vi "Error Handler.vi"(8 "error in (no error)":errorcluster, 9 "Motor Error Status (none)":T1, 10 "Error? (no error)":bool, 11 "Error type":u16(ring) items=["Default (no error)", "Scan timeout", "Invalid motor checksum", "Unexpected return string", "Invalid address range"]) -> (0 "error out":errorcluster)   [LabVIEW 2012, in "Roboteq.lvlib"]
doc: "This VI defines the error codes used for the Dynamixel motor driver."
uses:
  Roboteq.lvlib
  <instrlib>/Dynamixel Motor/Public/Motor Operation/Low Level/Alarm Setting.ctl
  <instrlib>/Dynamixel Motor/Dynamixel Motor.lvlib
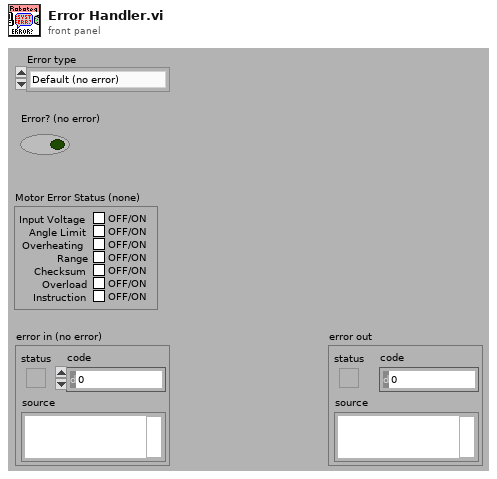
[diagram p1: front panel]
types:
  T1 = typedef "Dynamixel Motor.lvlib/Alarm Setting.ctl" = cluster{"Input Voltage":bool, "Angle Limit":bool, "Overheating ":bool, "Range":bool, "Checksum":bool, "Overload":bool, "Instruction":bool}
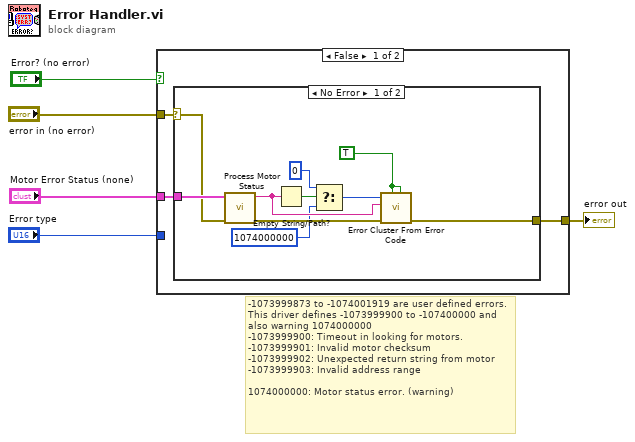
[diagram p0: block diagram]
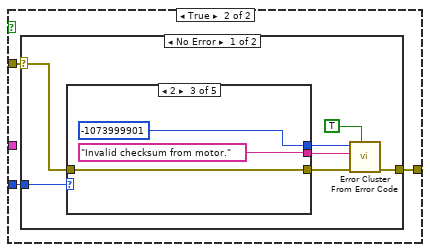
[diagram p3: hidden frame]
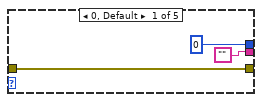
[diagram p4: hidden frame]
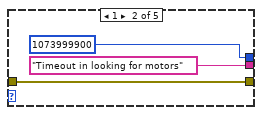
[diagram p5: hidden frame]
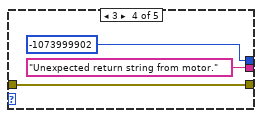
[diagram p6: hidden frame]
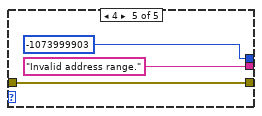
[diagram p7: hidden frame]
diagram:
  # "-1073999873 to -1074001919 are user defined errors.  This driver defines -1073999900 to -107400000 and also warning 1074000000\n-1073999900: Timeout in looking for motors.\n-1073999901: Invalid motor checksum\n-1073999902: Unexpected return string from motor\n-1073999903: Invalid address range\n\n1074000000: Motor status error. (warning)"
  n1 = case shown="False" "Error? (no error)" {
    tunnel: "error in (no error)" -> [w8 w22]
    tunnel: [w7 w21] -> w4
    tunnel: "Error type" -> [_ w20]
    tunnel: "Motor Error Status (none)" -> [w6 _]
    frame False {
      n2 = case shown="No Error" w8 {
        selector: w8 -> [w14 w19]
        tunnel: [w18 w19] -> w7
        tunnel: w6 -> [w16 _]
        frame No Error {
          w9 = TRUE ("show call chain? (False)")
          n3 = call "Process Motor Status.vi"("error in (no error)"=w14, "Motor Error Status"=w16) -> ("error out"=w13:errorcluster, "Error description"=w17:string)  [unwired: 8 in]
          n4 = Empty String/Path?(string/path=w17) -> (empty?=w12:bool)
          n5 = Select(t=0 ("y"), s=w12, f=1074000000 ("y")) -> (s? t:f=w15:i32)
          n6 = call <vilib>:"Error Cluster From Error Code.vi"("is warning? (False)"=w9, "show call chain? (False)"=w9, "error in (no error)"=w13, "error message (\"\")"=w17, "error code (0)"=w15) -> ("error out"=w18:errorcluster)  [unwired: 4 in]
        }
        frame Error {
        }
      }
    }
    frame True {
      n7 = case shown="No Error" w22 {
        selector: w22 -> [w26 w45]
        tunnel: [w29 w45] -> w21
        tunnel: w20 -> [w24 _]
        frame No Error {
          n8 = case shown="2" w24 {
            tunnel: ["" "Timeout in looking for motors" ("source") "Invalid checksum from motor." ("source") "Unexpected return string from motor." ("source") "Invalid address range." ("source")] -> w28
            tunnel: [0 ("y") 1073999900 ("y") -1073999901 ("y") -1073999902 ("y") -1073999903 ("y")] -> w27
            tunnel: w26 -> [w32 w33 w36 w39 w42]
            tunnel: [w32 w33 w36 w39 w42] -> w25
            frame 0, Default {
            }
            frame 1 {
            }
            frame 2 {
            }
            frame 3 {
            }
            frame 4 {
            }
          }
          n9 = call <vilib>:"Error Cluster From Error Code.vi"("show call chain? (False)"=TRUE, "error in (no error)"=w25, "error message (\"\")"=w28, "error code (0)"=w27) -> ("error out"=w29:errorcluster)  [unwired: 5 in]
        }
        frame Error {
        }
      }
    }
  }
  "error out" <- w4
